vi "Create_sweep_files.vi"(11 "Measurement File":path) -> (1 "Path 3":path, 2 "Path 2":path, 3 "Path":path)   [LabVIEW 2015]
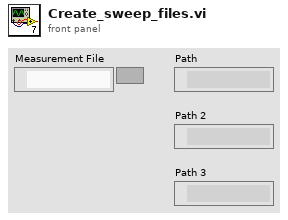
[diagram p1: front panel]
types:
  T1 = enum16{"open", "replace", "create", "open or create", "replace or create", "replace or create with confirmation"}
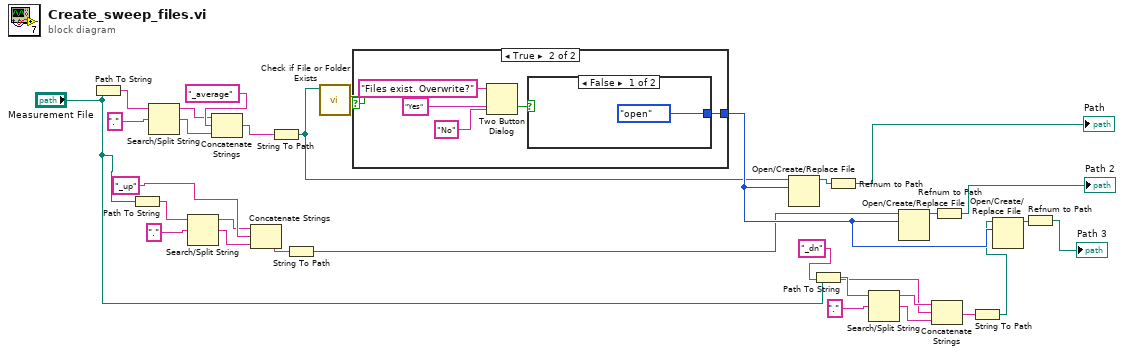
[diagram p0: block diagram]
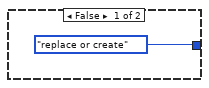
[diagram p2: hidden frame]
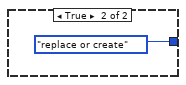
[diagram p3: hidden frame]
diagram:
  n1 = Path To String(path="Measurement File") -> (string=w5:string)
  n2 = Path To String(path="Measurement File") -> (string=w12:string)
  n3 = Search/Split String(string=w5, search string/char (-)=".") -> (substring before match=w7:string, match + rest of string=w28:string)  [unwired: 1 in, 1 out]
  n4 = Search/Split String(string=w12, search string/char (-)=".") -> (substring before match=w10:string, match + rest of string=w8:string)  [unwired: 1 in, 1 out]
  n5 = Concatenate Strings(w7, "_average" ("string"), w28) -> (w4:string)
  n6 = Concatenate Strings(w10, "_up" ("string"), w8) -> (w9:string)
  n7 = String To Path(string=w4) -> (path=w2:path)
  n8 = String To Path(string=w9) -> (path=w20:path)
  n9 = call <vilib>:"Check if File or Folder Exists.vi"("path"=w2) -> ("file or folder exists?"=w1:bool)  [unwired: 8 in, 2 out]
  n10 = case shown="True" w1 {
    tunnel: [T1."replace or create" ("operation (0:open)") w36] -> w22
    frame False {
    }
    frame True {
      n11 = Two Button Dialog(message="Files exist. Overwrite?", 1:"No" ("F button name (\"Cancel\")"), 2:"Yes" ("T button name (\"OK\")")) -> (T button?=w35:bool)
      n12 = case shown="False" w35 {
        tunnel: [T1."open" ("operation (0:open)") T1."replace or create" ("operation (0:open)")] -> w36
        frame False {
        }
        frame True {
        }
      }
    }
  }
  n13 = Open/Create/Replace File(file path (use dialog)=w2, operation (0:open)=w22) -> (refnum out=w3:refnum<file>)  [unwired: 4 in, 2 out]
  n14 = Path To String(path="Measurement File") -> (string=w15:string)
  n15 = Refnum to Path(1:w3) -> (0:→"Path":path)
  n16 = Search/Split String(string=w15, search string/char (-)=".") -> (substring before match=w17:string, match + rest of string=w19:string)  [unwired: 1 in, 1 out]
  n17 = Open/Create/Replace File(file path (use dialog)=w20, operation (0:open)=w22) -> (refnum out=w23:refnum<file>)  [unwired: 4 in, 2 out]
  n18 = Concatenate Strings(w17, "_dn" ("string"), w19) -> (w18:string)
  n19 = Refnum to Path(1:w23) -> (0:→"Path 2":path)
  n20 = String To Path(string=w18) -> (path=w21:path)
  n21 = Open/Create/Replace File(file path (use dialog)=w21, operation (0:open)=w22) -> (refnum out=w24:refnum<file>)  [unwired: 4 in, 2 out]
  n22 = Refnum to Path(1:w24) -> (0:→"Path 3":path)
